vi "cRIO_v1.vi"() -> ()   [LabVIEW 2015]
uses:
  <vilib>/FPGAPlugInAG/cRIO-9113/niLvFpga_Open_cRIO-9113.vi
  <vilib>/rvi/interface/common/dynamic/niFpgaDynamicAddResources.vi
  <vilib>/Utility/error.llb/Error Cluster From Error Code.vi
  <vilib>/FPGAPlugInAG/Dynamic/niLvFpga_Run_Dynamic.vi
  <vilib>/rvi/interface/common/niFpgaWaitOnOcc.vi
  <vilib>/rvi/errors/niLvFpgaAdjustHostInterfaceError.vi
  <vilib>/FPGAPlugInAG/Dynamic/niLvFpga_Close_Dynamic.vi
  <vilib>/rvi/interface/nirviOpenFPGA/nirviOpenFPGA.xnode
  FPGA Bitfiles/DW40ticks_FPGATarget_Fpgav1_TswWCJdvjoM.lvbitx
  <vilib>/rvi/interface/nirviMethod/nirviMethod.xnode
  <vilib>/rvi/interface/nirviReadWriteControl/nirviReadWriteControl.xnode
  <vilib>/rvi/interface/nirviCloseFPGA/nirviCloseFPGA.xnode
  <vilib>/rvi/errors/niLvFpgaMergeErrorWithErrorCode.vi
  <vilib>/FPGAPlugInAG/Dynamic/niLvFpga_ReadFifo_Dynamic.vi
  <vilib>/rvi/interface/Simulation/niFpgaSimulationCallBeginRW.vi
  <vilib>/FPGAPlugInAG/Dynamic/niLvFpga_StartFifo_Dynamic.vi
  <vilib>/FPGAPlugInAG/Dynamic/niLvFpga_ConfigureFifo_Dynamic.vi
  NiFpgaLv.dll
panel:
  out "Time(ms) for a loop":u32
  in  "datachanel":bool
  in  "Data write ON/OFF":bool
  out "backlog (Elements remaing on the write)":u32
  out "error out":errorcluster
  out "Actual Depth of FIFO":u32
  out "Initial write Elements Remaining":u32
  in  "stop":bool
  out "Timed Out?":bool
  out "Number of times timed out":u8
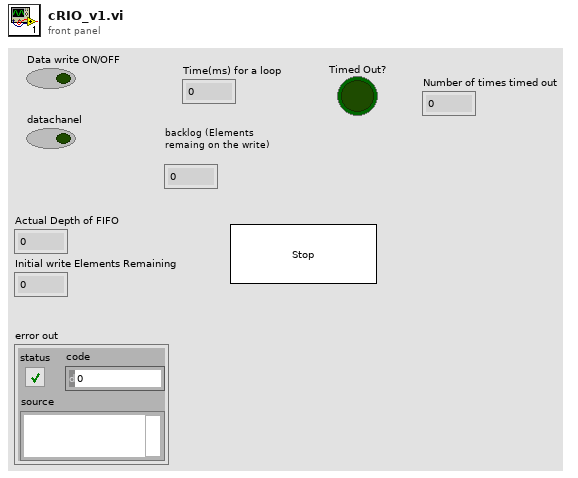
[diagram p1: front panel]
types:
  T1 = enum16{"open", "open or create", "create or replace", "create", "open (read-only)"}
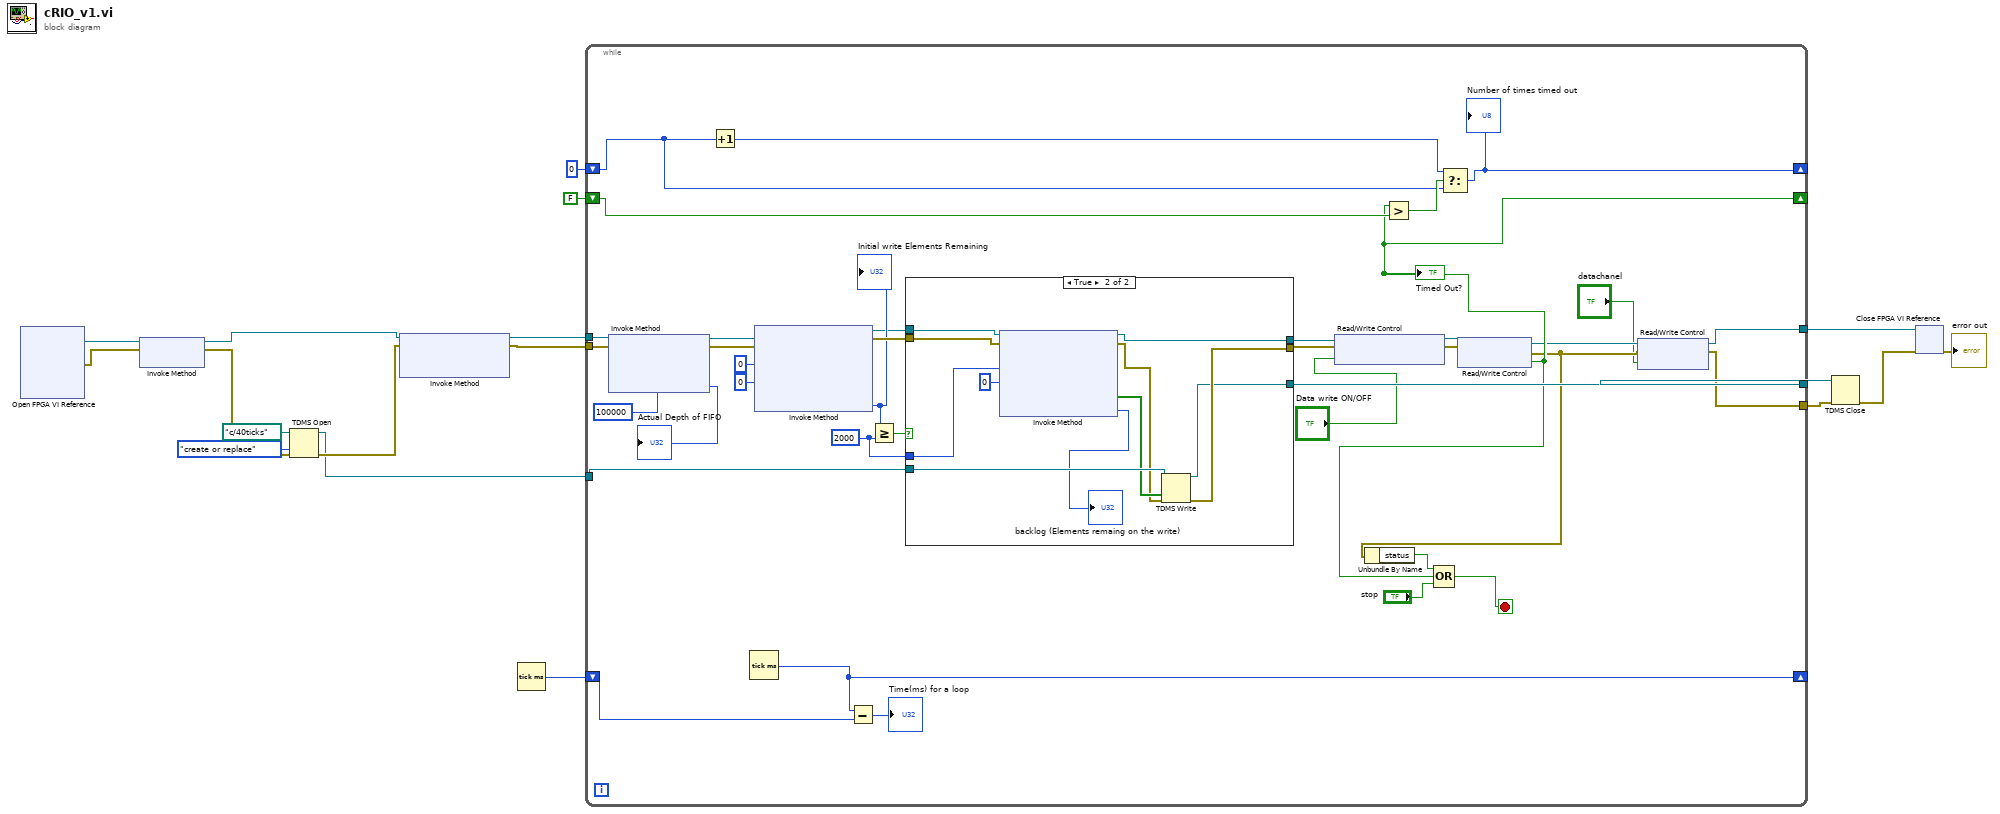
[diagram p0: block diagram]
diagram:
  n1 = xnode "Open FPGA VI Reference"() -> ("FPGA VI Reference Out"=w5:refnum<k20>, "error out"=w4:errorcluster)  [unwired: 2 in]
  n2 = xnode "Invoke Method"("FPGA VI Reference In"=w5, "error in"=w4) -> ("FPGA VI Reference Out"=w17:refnum<k20>, "error out"=w18:errorcluster)
  n3 = TDMS Open(8:w18, 10:T1."create or replace" ("operation (0:open)"), 11:path "c:/40ticks" ("file path")) -> (0:w16:errorcluster, 3:w11:refnum<k34>)  [unwired: 4 in]
  n4 = xnode "Invoke Method"("FPGA VI Reference In"=w17, "error in"=w16) -> ("FPGA VI Reference Out"=w15:refnum<k20>, "error out"=w14:errorcluster)  [unwired: 1 in]
  n5 = Tick Count (ms)() -> (millisecond timer value=w1:u32)
  n6 = while {
    tunnel: w15 -> [w55]
    tunnel: w14 -> [w54]
    tunnel: w11 -> [w46]
    tunnel: [w44] -> w9
    shift-right: [w27] -> _
    shift-left: FALSE ("Timed Out?") -> [w42]
    shift-right: [w38] -> _
    shift-left: u8 0 -> [w40]
    tunnel: [w24] -> w3
    tunnel: [w23] -> w2
    shift-right: [w20] -> _
    shift-left: w1 -> [w21]
    stop <- w43 stop-if-true
    w33 = u32 2000 ("y")
    n7 = xnode "Invoke Method"("FPGA VI Reference In"=w55, "error in"=w54, "Requested Depth"=u32 100000) -> ("FPGA VI Reference Out"=w51:refnum<k20>, "error out"=w50:errorcluster, "Actual Depth"=→"Actual Depth of FIFO":u32)
    n8 = Increment(x=w40) -> (x+1=w39:u8)
    n9 = Tick Count (ms)() -> (millisecond timer value=w20:u32)
    n10 = xnode "Invoke Method"("FPGA VI Reference In"=w51, "error in"=w50, "Number of Elements"=u32 0, "Timeout (ms)"=0) -> ("FPGA VI Reference Out"=w34:refnum<k20>, "error out"=w47:errorcluster, "Elements Remaining"=w35:u32)  [unwired: 1 out]
    "Initial write Elements Remaining" <- w35
    n11 = Subtract(x=w20, y=w21) -> (x-y=→"Time(ms) for a loop":u32)
    n12 = Greater Or Equal?(x=w35, y=w33) -> (x >= y?=w36:bool)
    n13 = case shown="True" w36 {
      tunnel: w47 -> [w56 w65]
      tunnel: w46 -> [w58 w69]
      tunnel: [w56 w68] -> w31
      tunnel: [w58 w67] -> w44
      tunnel: w34 -> [w57 w66]
      tunnel: [w57 w64] -> w32
      tunnel: w33 -> [_ w61]
      frame False {
      }
      frame True {
        n14 = xnode "Invoke Method"("FPGA VI Reference In"=w66, "error in"=w65, "Number of Elements"=w61, "Timeout (ms)"=0) -> ("FPGA VI Reference Out"=w64:refnum<k20>, "error out"=w62:errorcluster, "Data"=w63:bool[], "Elements Remaining"=→"backlog (Elements remaing on the write)":u32)
        n15 = TDMS Write(0:w69, 9:w63, 11:w62) -> (4:w67:refnum<k34>, 15:w68:errorcluster)  [unwired: 3 in, 2 out]
      }
    }
    n16 = xnode "Read/Write Control"("FPGA VI Reference In"=w32, "error in"=w31, "Data write ON/OFF"="Data write ON/OFF") -> ("FPGA VI Reference Out"=w30:refnum<k20>, "error out"=w29:errorcluster)
    n17 = xnode "Read/Write Control"("FPGA VI Reference In"=w30, "error in"=w29) -> ("FPGA VI Reference Out"=w26:refnum<k20>, "error out"=w25:errorcluster, "Timed Out?"=w27:bool)
    "Timed Out?" <- w27
    n18 = Unbundle By Name(w25) -> ("status"=w37:bool)
    n19 = Greater?(x=w27, y=w42) -> (0:w41:bool)
    n20 = Compound Arithmetic op=OR(w37, w27, "stop") -> (w43:bool)
    n21 = Select(t=w39, s=w41, f=w40) -> (s? t:f=w38:u8)
    "Number of times timed out" <- w38
    n22 = xnode "Read/Write Control"("FPGA VI Reference In"=w26, "error in"=w25, "datachanel"="datachanel") -> ("FPGA VI Reference Out"=w24:refnum<k20>, "error out"=w23:errorcluster)
  }
  n23 = TDMS Close(8:w2, 11:w9) -> (0:w10:errorcluster)  [unwired: 1 out]
  n24 = xnode "Close FPGA VI Reference"("FPGA VI Reference In"=w3, "error in"=w10) -> ("error out"=→"error out":errorcluster)
